vi "test_F9P.vi"() -> ()   [LabVIEW 2019] (continued)
17,042,38,25,01,241,,7*7D\r\n$GAGSV,3,3,09,36,35,314,34,7*48\r\n$GAGSV,3,1,09,02,04,287,,04,68,085,36,09,44,196,34,11,78,037,34,2*78\r\n$GAGSV,3,2,09,12,32,115,26,18,55,284,45,19,17,042,32,25,01,241,,2*73\r\n$GAGSV,3,3,09,36,35,314,40,2*4E\r\n$GBGSV,4,1,13,04,35,133,,05,09,257,,06,27,182,,07,09,201,,1*7B\r\n$GBGSV,4,2,13,08,65,355,41,09,07,194,,10,16,222,22,11,37,142,,1*7A\r\n$GBGSV,4,3,13,13,50,315,38,14,76,037,44,28,59,310,40,33,73,239,42,1*72\r\n$GBGSV,4,4,13,34,13,142,,1*46\r\n$GBGSV,4,1,13,04,35,133,,05,09,257,,06,27,182,,07,09,201,,3*79\r\n$GBGSV,4,2,13,08,65,355,37,09,07,194,,10,16,222,20,11,37,142,,3*7B\r\n$GBGSV,4,3,13,13,50,315,35,14,76,037,41,28,59,310,,33,73,239,,3*7A\r\n$GBGSV,4,4,13,34,13,142,,3*44\r\n$GNGLL,3723.62075,N,12656.98429,E,064340.00,A,A*79\r\n$GNRMC,064341.00,A,3723.62092,N,12656.98521,E,2.726,71.42,250720,,,A,V*36\r\n$GNVTG,71.42,T,,M,2.726,N,5.048,K,A*1B\r\n$GNGGA,064341.00,3723.62092,N,12656.98521,E,1,12,0.63,43.1,M,18.5,M,,*71\r\n$GNGSA,A,3,17,19,06,12,05,02,09,,,,,,1.10,0.63,0.90,1*08\r\n$GNGSA,A,3,85,70,71,72,,,,,,,,,1.10,0.63,0.90,2*07\r\n$GNGSA,A,3,36,19,11,04,09,12,,,,,,,1.10,0.63,0.90,3*0C\r\n$GNGSA,A,3,28,11,14,13,33,08,10,,,,,,1.10,0.63,0.90,4*0C\r\n$GPGSV,4,1,13,02,66,335,41,04,08,037,41,05,48,262,43,06,58,077,45,1*6E\r\n$GPGSV,4,2,13,07,06,104,22,09,38,057,41,12,18,262,22,13,09,191,20,1*6D\r\n$GPGSV,4,3,13,17,18,158,27,19,37,162,30,25,11,294,22,29,07,323,17,1*6D\r\n$GPGSV,4,4,13,30,01,134,,1*52\r\n$GPGSV,4,1,13,02,66,335,,04,08,037,30,05,48,262,39,06,58,077,37,6*62\r\n$GPGSV,4,2,13,07,06,104,,09,38,057,38,12,18,262,17,13,09,191,,6*60\r\n$GPGSV,4,3,13,17,18,158,26,19,37,162,,25,11,294,21,29,07,323,18,6*64\r\n$GPGSV,4,4,13,30,01,134,,6*55\r\n$GLGSV,2,1,06,70,54,030,36,71,69,224,42,72,18,217,29,84,08,134,10,1*76\r\n$GLGSV,2,2,06,85,63,113,43,86,52,337,,1*7C\r\n$GLGSV,2,1,06,70,54,030,,71,69,224,26,72,18,217,19,84,08,134,16,3*76\r\n$GLGSV,2,2,06,85,63,113,26,86,52,337,,3*7D\r\n$GAGSV,3,1,09,02,04,287,09,04,68,085,43,09,44,196,32,11,78,037,39,7*7D\r\n$GAGSV,3,2,09,12,32,115,33,18,55,284,41,19,17,042,44,25,01,241,,7*77\r\n$GAGSV,3,3,09,36,35,314,34,7*48\r\n$GAGSV,3,1,09,02,04,287,,04,68,085,40,09,44,196,33,11,78,037,34,2*7E\r\n$GAGSV,3,2,09,12,32,115,25,18,55,284,41,19,17,042,35,25,01,241,,2*73\r\n$GAGSV,3,3,09,36,35,314,31,2*48\r\n$GBGSV,4,1,13,04,35,133,,05,09,257,,06,27,182,,07,09,201,,1*7B\r\n$GBGSV,4,2,13,08,65,355,40,09,07,194,,10,16,222,22,11,37,142,,1*7B\r\n$GBGSV,4,3,13,13,50,315,36,14,76,037,43,28,59,310,38,33,73,239,41,1*77\r\n$GBGSV,4,4,13,34,13,142,,1*46\r\n$GBGSV,4,1,13,04,35,133,,05,09,257,,06,27,182,,07,09,201,,3*79\r\n$GBGSV,4,2,13,08,65,355,36,09,07,194,,10,16,222,20,11,37,142,30,3*79\r\n$GBGSV,4,3,13,13,50,315,33,14,76,037,40,28,59,310,,33,73,239,,3*7D\r\n$GBGSV,4,4,13,34,13,142,,3*44\r\n$GNGLL,3723.62092,N,12656.98521,E,064341.00,A,A*78\r\n$GNRMC,064342.00,A,3723.62115,N,12656.98619,E,3.064,70.18,250720,,,A,V*3D\r\n$GNVTG,70.18,T,,M,3.064,N,5.675,K,A*1D\r\n$GNGGA,064342.00,3723.62115,N,12656.98619,E,1,12,0.62,43.0,M,18.5,M,,*74\r\n$GNGSA,A,3,17,19,06,12,05,02,09,,,,,,1.07,0.62,0.87,1*09\r\n$GNGSA,A,3,85,70,71,72,,,,,,,,,1.07,0.62,0.87,2*06\r\n$GNGSA,A,3,36,19,11,04,09,12,,,,,,,1.07,0.62,0.87,3*0D\r\n$GNGSA,A,3,28,11,14,13,33,08,10,,,,,,1.07,0.62,0.87,4*0D\r\n$GPGSV,4,1,13,02,66,335,43,04,08,037,40,05,48,262,44,06,58,077,45,1*6A\r\n$GPGSV,4,2,13,07,06,104,,09,38,057,46,12,18,262,30,13,09,191,20,1*69\r\n$GPGSV,4,3,13,17,18,158,30,19,37,162,29,25,11,294,20,29,07,323,17,1*61\r\n$GPGSV,4,4,13,30,01,134,,1*52\r\n$GPGSV,4,1,13,02,66,335,,04,08,037,30,05,48,262,33,06,58,077,39,6*66\r\n$GPGSV,4,2,13,07,06,104,,09,38,057,37,12,18,262,16,13,09,191,,6*6E\r\n$GPGSV,4,3,13,17,18,158,25,19,37,162,,25,11,294,19,29,07,323,,6*65\r\n$GPGSV,4,4,13,30,01,134,,6*55\r\n$GLGSV,2,1,06,70,54,030,34,71,69,224,43,72,18,217,28,84,08,134,12,1*76\r\n$GLGSV,2,2,06,85,63,113,35,86,52,337,,1*7D\r\n$GLGSV,2,1,06,70,54,030,,71,69,224,26,72,18,217,19,84,08,134,16,3*76\r\n$GLGSV,2,2,06,85,63,113,26,86,52,337,,3*7D\r\n$GAGSV,3,1,09,02,04,287,11,04,68,085,42,09,44,196,36,11,78,037,39,7*71\r\n$GAGSV,3,2,09,12,32,115,30,18,55,284,39,19,17,042,44,25,01,241,,7*7B\r\n$GAGSV,3,3,09,36,35,314,33,7*4F\r\n$GAGSV,3,1,09,02,04,287,,04,68,085,37,09,44,196,32,11,78,037,30,2*7B\r\n$GAGSV,3,2,09,12,32,115,24,18,55,284,41,19,17,042,32,25,01,241,,2*75\r\n$GAGSV,3,3,09,36,35,314,25,2*4D\r\n$GBGSV,4,1,13,04,35,133,,05,09,257,,06,27,182,,07,09,201,,1*7B\r\n$GBGSV,4,2,13,08,65,355,42,09,07,194,,10,16,222,21,11,37,142,,1*7A\r\n$GBGSV,4,3,13,13,50,315,33,14,76,037,43,28,59,310,40,33,73,239,41,1*7D\r\n$GBGSV,4,4,13,34,13,142,,1*46\r\n$GBGSV,4,1,13,04,35,133,,05,09,257,,06,27,182,,07,09,201,,3*79\r\n$GBGSV,4,2,13,08,65,355,38,09,07,194,,10,16,222,19,11,37,142,29,3*75\r\n$GBGSV,4,3,13,13,50,315,37,14,76,037,36,28,59,310,,33,73,239,,3*78\r\n$GBGSV,4,4,13,34,13,142,,3*44\r\n$GNGLL,3723.62115,N,12656.98619,E,064342.00,A,A*7D\r\n$GNRMC,064343.00,A,3723.62142,N,12656.98714,E,2.933,68.12,250720,,,A,V*3B\r\n$GNVTG,68.12,T,,M,2.933,N,5.432,K,A*15\r\n$GNGGA,064343.00,3723.62142,N,12656.98714,E,1,12,0.62,42.9,M,18.5,M,,*73\r\n$GNGSA,A,3,17,19,06,12,05,02,09,,,,,,1.09,0.62,0.90,1*01\r\n$GNGSA,A,3,85,70,71,72,,,,,,,,,1.09,0.62,0.90,2*0E\r\n$GNGSA,A,3,36,19,11,04,09,12,,,,,,,1.09,0.62,0.90,3*05\r\n$GNGSA,A,3,28,11,14,13,33,08,10,,,,,,1.09,0.62,0.90,4*05\r\n$GPGSV,4,1,13,02,66,335,43,04,08,037,38,05,48,262,38,06,58,077,44,1*6F\r\n$GPGSV,4,2,13,07,06,104,,09,38,057,44,12,18,262,,13,09,191,22,1*6A\r\n$GPGSV,4,3,13,17,18,158,34,19,37,162,30,25,11,294,22,29,07,323,17,1*6F\r\n$GPGSV,4,4,13,30,01,134,,1*52\r\n$GPGSV,4,1,13,02,66,335,,04,08,037,30,05,48,262,38,06,58,077,35,6*61\r\n$GPGSV,4,2,13,07,06,104,,09,38,057,37,12,18,262,16,13,09,191,,6*6E\r\n$GPGSV,4,3,13,17,18,158,24,19,37,162,,25,11,294,17,29,07,323,,6*6A\r\n$GPGSV,4,4,13,30,01,134,,6*55\r\n$GLGSV,2,1,06,70,54,030,29,71,69,224,43,72,18,217,28,84,08,134,11,1*79\r\n$GLGSV,2,2,06,85,63,113,37,86,52,337,,1*7F\r\n$GLGSV,2,1,06,70,54,030,,71,69,224,27,72,18,217,18,84,08,134,16,3*76\r\n$GLGSV,2,2,06,85,63,113,26,86,52,337,,3*7D\r\n$GAGSV,3,1,09,02,04,287,06,04,68,085,41,09,44,196,38,11,78,037,40,7*74\r\n$GAGSV,3,2,09,12,32,115,34,18,55,284,38,19,17,042,43,25,01,241,,7*79\r\n$GAGSV,3,3,09,36,35,314,39,7*45\r\n$GAGSV,3,1,09,02,04,287,,04,68,085,33,09,44,196,35,11,78,037,34,2*7C\r\n$GAGSV,3,2,09,12,32,115,25,18,55,284,43,19,17,042,32,25,01,241,,2*76\r\n$GAGSV,3,3,09,36,35,314,35,2*4C\r\n$GBGSV,4,1,13,04,35,133,,05,09,257,,06,27,182,,07,09,201,,1*7B\r\n$GBGSV,4,2,13,08,65,355,41,09,07,194,,10,16,222,19,11,37,142,,1*72\r\n$GBGSV,4,3,13,13,50,315,37,14,76,037,44,28,59,310,38,33,73,239,41,1*71\r\n$GBGSV,4,4,13,34,13,142,,1*46\r\n$GBGSV,4,1,13,04,35,133,,05,09,257,,06,27,182,,07,09,201,,3*79\r\n$GBGSV,4,2,13,08,65,355,34,09,07,194,,10,16,222,21,11,37,142,32,3*78\r\n$GBGSV,4,3,13,13,50,315,33,14,76,037,43,28,59,310,,33,73,239,,3*7E\r\n$GBGSV,4,4,13,34,13,142,,3*44\r\n$GNGLL,3723.62142,N,12656.98714,E,064343.00,A,A*72\r\n$GNRMC,064344.00,A,3723.62178,N,12656.98806,E,2.945,64.77,250720,,,A,V*37\r\n$GNVTG,64.77,T,,M,2.945,N,5.453,K,A*1C\r\n$GNGGA,064344.00,3723.62178,N,12656.98806,E,1,12,0.62,42.9,M,18.5,M,,*71\r\n$GNGSA,A,3,17,19,06,12,05,02,09,,,,,,1.09,0.62,0.90,1*01\r\n$GNGSA,A,3,85,70,71,72,,,,,,,,,1.09,0.62,0.90,2*0E\r\n$GNGSA,A,3,36,19,11,04,09,12,,,,,,,1.09,0.62,0.90,3*05\r\n$GNGSA,A,3,28,11,14,13,33,08,10,,,,,,1.09,0.62,0.90,4*05\r\n$GPGSV,4,1,13,02,66,335,41,04,08,037,26,05,48,262,37,06,58,077,45,1*6C\r\n$GPGSV,4,2,13,07,06,104,,09,38,057,42,12,18,262,,13,09,191,25,1*6B\r\n$GPGSV,4,3,13,17,18,158,34,19,37,162,36,25,11,294,23,29,07,323,17,1*68\r\n$GPGSV,4,4,13,30,01,134,,1*52\r\n$GPGSV,4,1,13,02,66,335,,04,08,037,29,05,48,262,39,06,58,077,34,6*69\r\n$GPGSV,4,2,13,07,06,104,,09,38,057,41,12,18,262,17,13,09,191,,6*6E\r\n$GPGSV,4,3,13,17,18,158,31,19,37,162,,25,11,294,17,29,07,323,,6*6E\r\n$GPGSV,4,4,13,30,01,134,,6*55\r\n$GLGSV,2,1,06,70,54,030,30,71,69,224,41,72,18,217,28,84,08,134,18,1*7A\r\n$GLGSV,2,2,06,85,63,113,37,86,52,337,,1*7F\r\n$GLGSV,2,1,06,70,54,030,,71,69,224,33,72,18,217,18,84,08,134,21,3*77\r\n$GLGSV,2,2,06,85,63,113,31,86,52,337,,3*7B\r\n$GAGSV,3,1,09,02,04,287,09,04,68,085,42,09,44,196,40,11,78,037,40,7*77\r\n$GAGSV,3,2,09,12,32,115,38,18,55,284,38,19,17,042,41,25,01,241,,7*77\r\n$GAGSV,3,3,09,36,35,314,39,7*45\r\n$GAGSV,3,1,09,02,04,287,,04,68,085,34,09,44,196,31,11,78,037,35,2*7E\r\n$GAGSV,3,2,09,12,32,115,25,18,55,284,42,19,17,042,35,25,01,241,,2*70\r\n$GAGSV,3,3,09,36,35,314,38,2*41\r\n$GBGSV,4,1,13,04,35,133,,05,09,257,,06,27,182,,07,09,201,,1*7B\r\n$GBGSV,4,2,13,08,65,355,39,09,07,194,,10,16,222,22,11,37,142,28,1*7F\r\n$GBGSV,4,3,13,13,50,315,37,14,76,037,43,28,59,310,42,33,73,239,42,1*78\r\n$GBGSV,4,4,13,34,13,142,,1*46\r\n$GBGSV,4,1,13,04,35,133,,05,09,257,,06,27,182,,07,09,201,,3*79\r\n$GBGSV,4,2,13,08,65,355,34,09,07,194,,10,16,222,21,11,37,142,29,3*72\r\n$GBGSV,4,3,13,13,50,315,38,14,76,037,42,28,59,310,,33,73,239,,3*74\r\n$GBGSV,4,4,13,34,13,142,,3*44\r\n$GNGLL,3723.62178,N,12656.98806,E,064344.00,A,A*70\r\n$GNRMC,064345.00,A,3723.62207,N,12656.98888,E,2.663,64.15,250720,,,A,V*34\r\n$GNVTG,64.15,T,,M,2.663,N,4.931,K,A*1B\r\n$GNGGA,064345.00,3723.62207,N,12656.98888,E,1,12,0.62,42.7,M,18.5,M,,*73\r\n$GNGSA,A,3,17,19,06,12,05,02,09,,,,,,1.09,0.62,0.90,1*01\r\n$GNGSA,A,3,85,70,71,72,,,,,,,,,1.09,0.62,0.90,2*0E\r\n$GNGSA,A,3,36,19,11,04,09,12,,,,,,,1.09,0.62,0.90,3*05\r\n$GNGSA,A,3,28,11,14,13,33,08,10,,,,,,1.09,0.62,0.90,4*05\r\n$GPGSV,4,1,13,02,66,335,43,04,08,037,25,05,48,262,40,06,58,077,47,1*6F\r\n$GPGSV,4,2,13,07,06,104,,09,38,057,44,12,18,262,,13,09,191,23,1*6B\r\n$GPGSV,4,3,13,17,18,158,35,19,37,162,29,25,11,294,,29,07,323,17,1*66\r\n$GPGSV,4,4,13,30,01,134,,1*52\r\n$GPGSV,4,1,13,02,66,335,,04,08,037,26,05,48,262,37,06,58,077,40,6*6B\r\n$GPGSV,4,2,13,07,06,104,,09,38,057,33,12,18,262,15,13,09,191,,6*69\r\n$GPGSV,4,3,13,17,18,158,31,19,37,162,,25,11,294,18,29,07,323,,6*61\r\n$GPGSV,4,4,13,30,01,134,,6*55\r\n$GLGSV,2,1,06,70,54,030,34,71,69,224,38,72,18,217,29,84,08,134,14,1*7D\r\n$GLGSV,2,2,06,85,63,113,31,86,52,337,,1*79\r\n$GLGSV,2,1,06,70,54,030,,71,69,224,29,72,18,217,,84,08,134,23,3*77\r\n$GLGSV,2,2,06,85,63,113,31,86,52,337,,3*7B\r\n$GAGSV,3,1,09,02,04,287,09,04,68,085,41,09,44,196,37,11,78,037,39,7*7A\r\n$GAGSV,3,2,09,12,32,115,32,18,55,284,37,19,17,042,40,25,01,241,,7*73\r\n$GAGSV,3,3,09,36,35,314,39,7*45\r\n$GAGSV,3,1,09,02,04,287,,04,68,085,36,09,44,196,31,11,78,037,31,2*78\r\n$GAGSV,3,2,09,12,32,115,25,18,55,284,41,19,17,042,35,25,01,241,,2*73\r\n$GAGSV,3,3,09,36,35,314,39,2*40\r\n$GBGSV,4,1,13,04,35,133,,05,09,257,,06,27,182,,07,09,201,,1*7B\r\n$GBGSV,4,2,13,08,65,355,41,09,07,194,,10,16,222,22,11,37,142,28,1*70\r\n$GBGSV,4,3,13,13,50,315,37,14,76,037,43,28,59,310,41,33,73,239,40,1*79\r\n$GBGSV,4,4,13,34,13,142,,1*46\r\n$GBGSV,4,1,13,04,35,133,,05,09,257,,06,27,182,,07,09,201,,3*79\r\n$GBGSV,4,2,13,08,65,355,38,09,07,194,,10,16,222,22,11,37,142,36,3*73\r\n$GBGSV,4,3,13,13,50,315,35,14,76,037,35,28,59,310,,33,73,239,,3*79\r\n$GBGSV,4,4,13,34,13,142,,3*44\r\n$GNGLL,3723.62207,N,12656.98888,E,064345.00,A,A*7C\r\n$GNRMC,064346.00,A,3723.62235,N,12656.98966,E,2.503,64.12,250720,,,A,V*35\r\n$GNVTG,64.12,T,,M,2.503,N,4.636,K,A*11\r\n$GNGGA,064346.00,3723.62235,N,12656.98966,E,1,12,0.66,42.3,M,18.5,M,,*70\r\n$GNGSA,A,3,17,19,06,05,02,09,,,,,,,1.18,0.66,0.98,1*0E\r\n$GNGSA,A,3,85,70,71,72,,,,,,,,,1.18,0.66,0.98,2*02\r\n$GNGSA,A,3,36,19,11,04,09,12,,,,,,,1.18,0.66,0.98,3*09\r\n$GNGSA,A,3,28,11,14,13,33,08,10,,,,,,1.18,0.66,0.98,4*09\r\n$GPGSV,4,1,13,02,66,335,42,04,08,037,35,05,48,262,40,06,58,077,45,1*6D\r\n$GPGSV,4,2,13,07,06,104,,09,38,057,47,12,18,262,27,13,09,191,21,1*6F\r\n$GPGSV,4,3,13,17,18,158,27,19,37,162,29,25,11,294,27,29,07,323,19,1*6E\r\n$GPGSV,4,4,13,30,01,134,,1*52\r\n$GPGSV,4,1,13,02,66,335,,04,08,037,24,05,48,262,36,06,58,077,39,6*66\r\n$GPGSV,4,2,13,07,06,104,,09,38,057,29,12,18,262,,13,09,191,,6*66\r\n$GPGSV,4,3,13,17,18,158,25,19,37,162,,25,11,294,18,29,07,323,,6*64\r\n$GPGSV,4,4,13,30,01,134,,6*55\r\n$GLGSV,2,1,06,70,54,030,30,71,69,224,38,72,18,217,27,84,08,134,16,1*75\r\n$GLGSV,2,2,06,85,63,113,33,86,52,337,,1*7B\r\n$GLGSV,2,1,06,70,54,030,,71,69,224,31,72,18,217,19,84,08,134,23,3*76\r\n$GLGSV,2,2,06,85,63,113,31,86,52,337,,3*7B\r\n$GAGSV,3,1,09,02,04,287,08,04,68,085,40,09,44,196,39,11,78,037,38,7*75\r\n$GAGSV,3,2,09,12,32,115,32,18,55,284,40,19,17,042,41,25,01,241,,7*72\r\n$GAGSV,3,3,09,36,35,314,39,7*45\r\n$GAGSV,3,1,09,02,04,287,,04,68,085,36,09,44,196,31,11,78,037,30,2*79\r\n$GAGSV,3,2,09,12,32,115,26,18,55,284,43,19,17,042,38,25,01,241,,2*7F\r\n$GAGSV,3,3,09,36,35,314,40,2*4E\r\n$GBGSV,4,1,13,04,35,133,,05,09,257,,06,27,182,,07,09,201,,1*7B\r\n$GBGSV,4,2,13,08,65,355,41,09,07,194,,10,16,222,20,11,37,142,32,1*79\r\n$GBGSV,4,3,13,13,50,315,38,14,76,037,43,28,59,310,42,33,73,239,39,1*7B\r\n$GBGSV,4,4,13,34,13,142,26,1*42\r\n$GBGSV,4,1,13,04,35,133,,05,09,257,,06,27,182,,07,09,201,,3*79\r\n$GBGSV,4,2,13,08,65,355,36,09,07,194,,10,16,222,23,11,37,142,38,3*72\r\n$GBGSV,4,3,13,13,50,315,35,14,76,037,37,28,59,310,,33,73,239,,3*7B\r\n$GBGSV,4,4,13,34,13,142,,3*44\r\n$GNGLL,3723.62235,N,12656.98966,E,064346.00,A,A*7F\r\n$GNRMC,064347.00,A,3723.62262,N,12656.99047,E,2.634,64.92,250720,,,A,V*32\r\n$GNVTG,64.92,T,,M,2.634,N,4.879,K,A*1B\r\n$GNGGA,064347.00,3723.62262,N,12656.99047,E,1,12,0.62,42.1,M,18.5,M,,*7E\r\n$GNGSA,A,3,17,19,06,12,05,02,09,,,,,,1.09,0.62,0.90,1*01\r\n$GNGSA,A,3,85,70,71,72,,,,,,,,,1.09,0.62,0.90,2*0E\r\n$GNGSA,A,3,36,19,11,04,09,12,,,,,,,1.09,0.62,0.90,3*05\r\n$GNGSA,A,3,28,11,14,13,33,34,08,10,,,,,1.09,0.62,0.90,4*02\r\n$GPGSV,4,1,13,02,66,335,44,04,08,037,27,05,48,262,42,06,58,077,46,1*69\r\n$GPGSV,4,2,13,07,06,104,,09,38,057,45,12,18,262,27,13,09,191,20,1*6C\r\n$GPGSV,4,3,13,17,18,158,26,19,37,162,30,25,11,293,26,29,07,323,19,1*61\r\n$GPGSV,4,4,13,30,01,134,,1*52\r\n$GPGSV,4,1,13,02,66,335,,04,08,037,24,05,48,262,38,06,58,077,36,6*67\r\n$GPGSV,4,2,13,07,06,104,,09,38,057,40,12,18,262,,13,09,191,,6*69\r\n$GPGSV,4,3,13,17,18,158,23,19,37,162,,25,11,293,18,29,07,323,23,6*64\r\n$GPGSV,4,4,13,30,01,134,,6*55\r\n$GLGSV,2,1,06,70,54,030,36,71,69,224,40,72,18,217,27,84,08,134,14,1*7E\r\n$GLGSV,2,2,06,85,63,113,37,86,52,337,,1*7F\r\n$GLGSV,2,1,06,70,54,030,,71,69,224,26,72,18,217,15,84,08,134,23,3*7C\r\n$GLGSV,2,2,06,85,63,113,22,86,52,337,,3*79\r\n$GAGSV,3,1,09,02,04,287,09,04,68,085,38,09,44,196,39,11,78,037,39,7*7A\r\n$GAGSV,3,2,09,12,32,115,28,18,55,284,39,19,17,042,38,25,01,241,,7*79\r\n$GAGSV,3,3,09,36,35,314,40,7*4B\r\n$GAGSV,3,1,09,02,04,287,,04,68,085,35,09,44,196,36,11,78,037,32,2*7F\r\n$GAGSV,3,2,09,12,32,115,25,18,55,284,43,19,17,042,38,25,01,241,,2*7C\r\n$GAGSV,3,3,09,36,35,314,38,2*41\r\n$GBGSV,4,1,13,04,35,133,,05,09,257,,06,27,182,,07,09,201,,1*7B\r\n$GBGSV,4,2,13,08,65,355,42,09,07,194,,10,16,222,20,11,37,142,27,1*7E\r\n$GBGSV,4,3,13,13,50,315,38,14,76,037,43,28,59,310,40,33,73,239,40,1*77\r\n$GBGSV,4,4,13,34,13,142,25,1*41\r\n$GBGSV,4,1,13,04,35,133,,05,09,257,,06,27,182,,07,09,201,,3*79\r\n$GBGSV,4,2,13,08,65,355,37,09,07,194,,10,16,222,23,11,37,142,35,3*7E\r\n$GBGSV,4,3,13,13,50,315,35,14,76,037,37,28,59,310,,33,73,239,,3*7B\r\n$GBGSV,4,4,13,34,13,142,,3*44\r\n$GNGLL,3723.62262,N,12656.99047,E,064347.00,A,A*77\r\n$GNRMC,064348.00,A,3723.62290,N,12656.99130,E,2.532,65.01,250720,,,A,V*3F\r\n$GNVTG,65.01,T,,M,2.532,N,4.689,K,A*14\r\n$GNGGA,064348.00,3723.62290,N,12656.99130,E,1,12,0.62,42.2,M,18.5,M,,*7E\r\n$GNGSA,A,3,17,19,06,12,05,02,09,,,,,,1.09,0.62,0.90,1*01\r\n$GNGSA,A,3,85,70,71,72,,,,,,,,,1.09,0.62,0.90,2*0E\r\n$GNGSA,A,3,36,19,11,04,09,12,,,,,,,1.09,0.62,0.90,3*05\r\n$GNGSA,A,3,28,11,14,13,33,08,10,,,,,,1.09,0.62,0.90,4*05\r\n$GPGSV,4,1,13,02,66,335,45,04,08,037,26,05,48,262,41,06,58,077,43,1*6F\r\n$GPGSV,4,2,13,07,06,104,21,09,38,057,45,12,18,262,28,13,09,191,19,1*6A\r\n$GPGSV,4,3,13,17,18,158,31,19,37,162,28,25,11,293,25,29,07,323,21,1*66\r\n$GPGSV,4,4,13,30,01,134,,1*52\r\n$GPGSV,4,1,13,02,66,335,,04,08,037,22,05,48,262,36,06,58,077,35,6*6C\r\n$GPGSV,4,2,13,07,06,104,,09,38,057,39,12,18,262,20,13,09,191,,6*65\r\n$GPGSV,4,3,13,17,18,158,23,19,37,162,,25,11,293,16,29,07,323,20,6*69\r\n$GPGSV,4,4,13,30,01,134,,6*55\r\n$GLGSV,2,1,06,70,54,030,33,71,69,224,39,72,18,217,26,84,08,134,10,1*70\r\n$GLGSV,2,2,06,85,63,113,29,86,52,337,,1*70\r\n$GLGSV,2,1,06,70,54,030,,71,69,224,27,72,18,217,17,84,08,134,21,3*7D\r\n$GLGSV,2,2,06,85,63,113,22,86,52,337,,3*79\r\n$GAGSV,3,1,09,02,04,287,07,04,68,085,38,09,44,196,40,11,78,037,37,7*74\r\n$GAGSV,3,2,09,12,32,115,27,18,55,284,41,19,17,042,28,25,01,241,,7*78\r\n$GAGSV,3,3,09,36,35,314,41,7*4A\r\n$GAGSV,3,1,09,02,04,287,,04,68,085,35,09,44,196,35,11,78,037,34,2*7A\r\n$GAGSV,3,2,09,12,32,115,25,18,55,284,44,19,17,042,36,25,01,241,,2*75\r\n$GAGSV,3,3,09,36,35,314,40,2*4E\r\n$GBGSV,4,1,13,04,35,133,,05,09,257,,06,27,182,,07,09,201,,1*7B\r\n$GBGSV,4,2,13,08,65,355,42,09,07,194,,10,16,222,18,11,37,142,30,1*73\r\n$GBGSV,4,3,13,13,50,315,41,14,76,037,43,28,59,310,35,33,73,239,42,1*79\r\n$GBGSV,4,4,13,34,13,142,,1*46\r\n$GBGSV,4,1,13,04,35,133,,05,09,257,,06,27,182,,07,09,201,,3*79\r\n$GBGSV,4,2,13,08,65,355,38,09,07,194,,10,16,222,20,11,37,142,35,3*72\r\n$GBGSV,4,3,13,13,50,315,38,14,76,037,37,28,59,310,,33,73,239,,3*76\r\n$GBGSV,4,4,13,34,13,142,,3*44\r\n$GNGLL,3723.62290,N,12656.99130,E,064348.00,A,A*74\r\n$GNRMC,064349.00,A,3723.62318,N,12656.99213,E,2.651,64.45,250720,,,A,V*3A\r\n$GNVTG,64.45,T,,M,2.651,N,4.909,K,A*14\r\n$GNGGA,064349.00,3723.62318,N,12656.99213,E,1,12,0.66,42.2,M,18.5,M,,*78\r\n$GNGSA,A,3,17,19,06,05,02,09,,,,,,,1.18,0.66,0.98,1*0E\r\n$GNGSA,A,3,85,70,71,72,,,,,,,,,1.18,0.66,0.98,2*02\r\n$GNGSA,A,3,36,19,11,04,09,12,,,,,,,1.18,0.66,0.98,3*09\r\n$GNGSA,A,3,28,11,14,13,33,08,10,,,,,,1.18,0.66,0.98,4*09\r\n$GPGSV,4,1,13,02,66,335,43,04,08,037,26,05,48,262,41,06,58,077,40,1*6A\r\n$GPGSV,4,2,13,07,06,104,22,09,38,057,46,12,18,262,,13,09,191,19,1*60\r\n$GPGSV,4,3,13,17,18,158,25,19,37,162,29,25,11,293,25,29,07,323,23,1*60\r\n$GPGSV,4,4,13,30,01,134,,1*52\r\n$GPGSV,4,1,13,02,66,335,,04,08,037,22,05,48,262,36,06,58,077,36,6*6F\r\n$GPGSV,4,2,13,07,06,104,,09,38,057,37,12,18,262,19,13,09,191,,6*61\r\n$GPGSV,4,3,13,17,18,158,22,19,37,162,,25,11,293,15,29,07,323,,6*69\r\n$GPGSV,4,4,13,30,01,134,,6*55\r\n$GLGSV,2,1,06,70,54,030,34,71,69,224,40,72,18,217,26,84,08,134,16,1*7F\r\n$GLGSV,2,2,06,85,63,113,28,86,52,337,,1*71\r\n$GLGSV,2,1,06,70,54,030,,71,69,224,32,72,18,217,28,84,08,134,20,3*74\r\n$GLGSV,2,2,06,85,63,113,22,86,52,337,,3*79\r\n$GAGSV,3,1,09,02,04,287,07,04,68,085,37,09,44,196,41,11,78,037,38,7*75\r\n$GAGSV,3,2,09,12,32,115,27,18,55,284,42,19,17,042,30,25,01,241,,7*72\r\n$GAGSV,3,3,09,36,35,314,41,7*4A\r\n$GAGSV,3,1,09,02,04,287,,04,68,085,27,09,44,196,33,11,78,037,30,2*7B\r\n$GAGSV,3,2,09,12,32,115,24,18,55,284,44,19,17,042,36,25,01,241,,2*74\r\n$GAGSV,3,3,09,36,35,314,36,2*4F\r\n$GBGSV,4,1,13,04,35,133,,05,09,257,,06,27,182,,07,09,201,,1*7B\r\n$GBGSV,4,2,13,08,65,355,42,09,07,194,,10,16,222,19,11,37,142,25,1*76\r\n$GBGSV,4,3,13,13,50,315,39,14,76,037,41,28,59,310,39,33,73,239,39,1*74\r\n$GBGSV,4,4,13,34,13,142,,1*46\r\n$GBGSV,4,1,13,04,35,133,,05,09,257,,06,27,182,,07,09,201,,3*79\r\n$GBGSV,4,2,13,08,65,355,38,09,07,194,,10,16,222,17,11,37,142,29,3*7B\r\n$GBGSV,4,3,13,13,50,315,35,14,76,037,37,28,59,310,,33,73,239,,3*7B\r\n$GBGSV,4,4,13,34,13,142,,3*44\r\n$GNGLL,3723.62318,N,12656.99213,E,064349.00,A,A*76\r\n$GNRMC,064350.00,A,3723.62348,N,12656.99296,E,2.568,63.77,250720,,,A,V*35\r\n$GNVTG,63.77,T,,M,2.568,N,4.756,K,A*1F\r\n$GNGGA,064350.00,3723.62348,N,12656.99296,E,1,12,0.61,42.1,M,18.5,M,,*7C\r\n$GNGSA,A,3,17,19,06,12,05,02,09,,,,,,1.06,0.61,0.87,1*0B\r\n$GNGSA,A,3,85,70,71,72,,,,,,,,,1.06,0.61,0.87,2*04\r\n$GNGSA,A,3,36,19,11,04,09,12,,,,,,,1.06,0.61,0.87,3*0F\r\n$GNGSA,A,3,28,11,14,13,33,08,10,,,,,,1.06,0.61,0.87,4*0F\r\n$GPGSV,4,1,13,02,66,335,44,04,08,037,26,05,48,262,40,06,58,077,40,1*6C\r\n$GPGSV,4,2,13,07,06,104,21,09,38,057,45,12,18,262,36,13,09,191,20,1*6F\r\n$GPGSV,4,3,13,17,18,158,26,19,37,162,32,25,11,293,26,29,07,323,23,1*6A\r\n$GPGSV,4,4,13
